vi "周期触发定时器.vi"(5 "time (ms)":u32, 9 "reset":bool) -> (6 "Triggered":bool, 8 "time since last call":u32, 10 "timer value":u32)   [LabVIEW 2012, in "毫秒定时器.lvlib"]
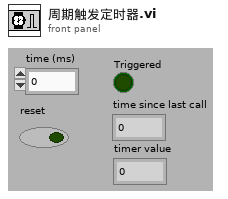
[diagram p1: front panel]
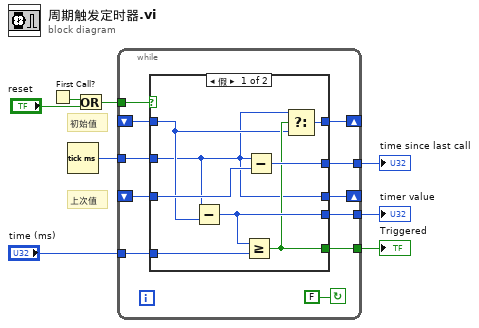
[diagram p0: block diagram]
diagram:
  # "初始值"
  # "上次值"
  n1 = First Call?() -> (First Call?: T/F=w6:bool)
  n2 = Tick Count (ms)() -> (millisecond timer value=w5:u32)
  n3 = Or(x=w6, y="reset") -> (x .or. y?=w8:bool)
  n4 = while {
    shift-left: _ -> [w10]
    shift-right: [w16] -> _
    shift-left: _ -> [w14]
    shift-right: [w15] -> _
    tunnel: w8 -> [w18]
    tunnel: w5 -> [w17]
    tunnel: "time (ms)" -> [w12]
    tunnel: [w13] -> w3
    tunnel: [w11] -> w2
    tunnel: [w9] -> w1
    stop <- FALSE continue-if-true
    n5 = case shown="假" w18 {
      tunnel: w17 -> [w20 w28]
      tunnel: [w20 w28] -> w16
      tunnel: [w23 w28] -> w15
      tunnel: w14 -> [w21 _]
      tunnel: [w27 _] -> w13
      tunnel: w12 -> [w26 _]
      tunnel: [w22 _] -> w11
      tunnel: w10 -> [w25 _]
      tunnel: [w24 _] -> w9
      frame False {
        n6 = Subtract(x=w20, y=w21) -> (x-y=w27:u32)
        n7 = Greater Or Equal?(x=w27, y=w26) -> (x >= y?=w22:bool)
        n8 = Subtract(x=w20, y=w25) -> (x-y=w24:u32)
        n9 = Select(t=w20, s=w22, f=w21) -> (s? t:f=w23:u32)
      }
      frame True {
      }
    }
  }
  "time since last call" <- w1
  "Triggered" <- w2
  "timer value" <- w3
